vi "Settings Requested Path.vi"() -> (3 "Requested Path":path)   [LabVIEW 2021]
uses:
  vi.lib/LabVIEW Icon API/lv_icon/lv_icon.lvlib
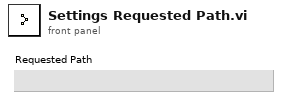
[diagram p1: front panel]
types:
  T1 = typedef "Who Invoked Icon Editor.ctl" = cluster{"Icon Editor Invoker Type":T2, "App Refnum of Invoker":refnum<vi>, "Qualified Name of Invoker":string, "Path to Invoker":path}
  T2 = typedef "Icon Editor Invoker Type.ctl" = enum32{"Unknown Icon Source", "VI Icon", "Library Icon (any library type)", "Palette icon", "Icon from App Method"}
  T3 = typedef "Pathes.ctl" = enum16{"Root Path", "Icon Templates", "Icon Templates VI", "Icon Templates Lib", "Glyphs"}
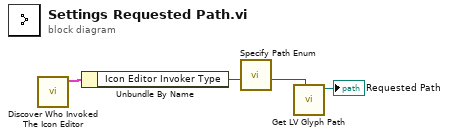
[diagram p0: block diagram]
diagram:
  n1 = call <resource>:"Discover Who Invoked The Icon Editor.vi"() -> ("Who Invoked The Icon Editor?"=w3:T1)  [unwired: 11 out]
  n2 = Unbundle By Name(w3) -> ("Icon Editor Invoker Type"=w2:T2)
  n3 = call "Specify Path Enum.vi"("Icon Editor Invoker Type"=w2) -> ("Path"=w4:T3)  [unwired: 10 out]
  n4 = call "Get LV Glyph Path.vi"("Path"=w4) -> ("Requested Path"=→"Requested Path":path)  [unwired: 2 in, 8 out]
